vi "Get Oscillator Amplitude Sweep Stop Amplitude.vi"(8 "error in (no error)":errorcluster, 11 "VISA resource name":refnum<visa-resource-name>) -> (0 "error out":errorcluster, 2 "Oscillator Amplitude Sweep Stop Amplitude (V)":dbl, 3 "VISA resource name out":refnum<visa-resource-name>)   [LabVIEW 2016, in "SR7270 Drivers.lvlib"]
uses:
  SR7270 Drivers.lvlib
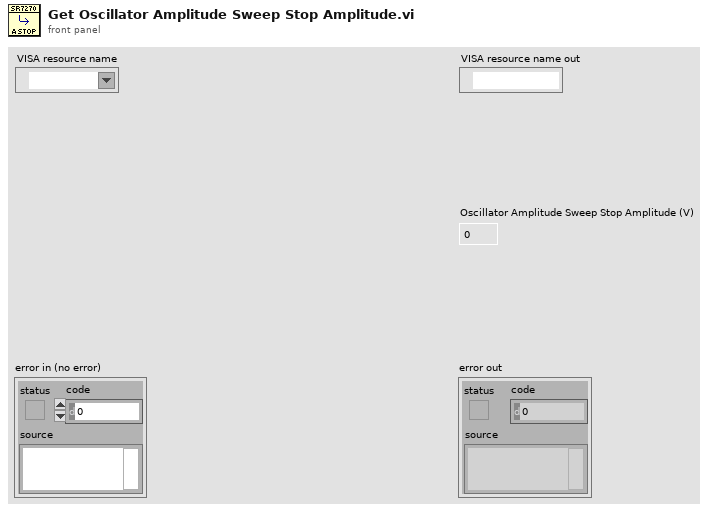
[diagram p1: front panel]
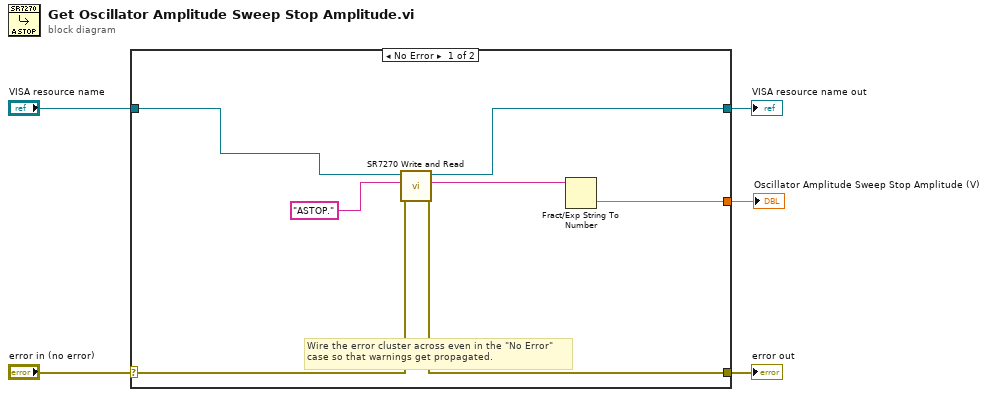
[diagram p0: block diagram]
diagram:
  n1 = case shown="No Error" "error in (no error)" {
    selector: "error in (no error)" -> [w12 w14]
    tunnel: [w11 w14] -> w4
    tunnel: [w6 w13] -> w2
    tunnel: "VISA resource name" -> [w7 w13]
    tunnel: [w8 _] -> w1
    frame No Error {
      # "Wire the error cluster across even in the \"No Error\"\ncase so that warnings get propagated."
      n2 = call "SR7270 Write and Read.vi"("error in (no error)"=w12, "Command Name"="ASTOP.", "VISA resource name"=w7) -> ("error out"=w11:errorcluster, "Read"=w9:string, "VISA resource name out"=w6:refnum<visa-resource-name>)  [unwired: 5 in, 1 out]
      n3 = Fract/Exp String To Number(string=w9) -> (number=w8:dbl)  [unwired: 3 in, 1 out]
    }
    frame Error {
    }
  }
  "error out" <- w4
  "VISA resource name out" <- w2
  "Oscillator Amplitude Sweep Stop Amplitude (V)" <- w1
